vi "Delete Project Tasks.vi"(8 "error in (no error)":errorcluster, 9 "Tasks":string[](array[string]), 10 "Project Name":string, 11 "Projects in":refnum<class "Projects.lvclass">) -> (0 "error out":errorcluster, 2 "Success?":bool, 3 "Projects out":refnum<class "Projects.lvclass">)   [LabVIEW 2020, in "Projects.lvclass"]
doc: "Removes the Tasks from project indicated by Project Name. Success? will output True if the tasks are not present in the Project and the Project Name was a valid name.\n\n03/2025 Erich Schlieper"
uses:
  Projects.lvclass
  Projects.lvclass/Projects.ctl
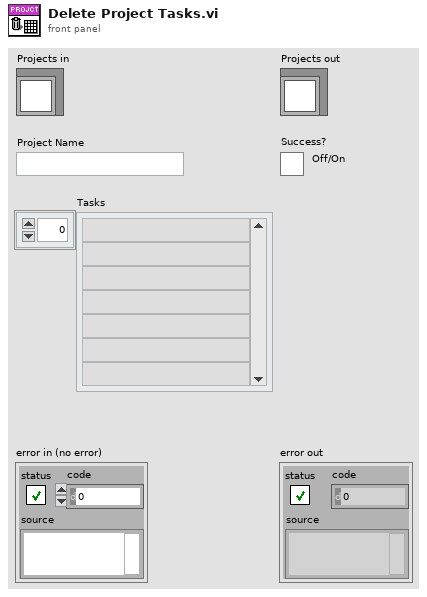
[diagram p1: front panel]
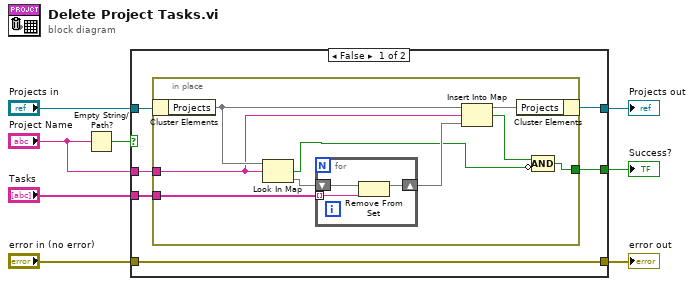
[diagram p0: block diagram]
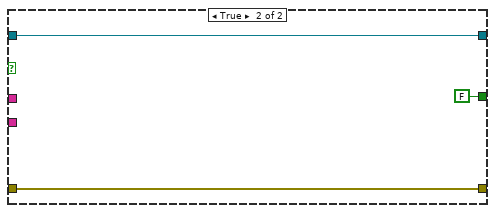
[diagram p2: hidden frame]
diagram:
  n1 = Empty String/Path?(string/path="Project Name") -> (empty?=w1:bool)
  n2 = case shown="False" w1 {
    tunnel: [w13 w29] -> w7
    tunnel: [w12 w28] -> w5
    tunnel: "Projects in" -> [w14 w28]
    tunnel: "Project Name" -> [w11 _]
    tunnel: "Tasks" -> [w10 _]
    tunnel: [w9 FALSE] -> w3
    tunnel: "error in (no error)" -> [w13 w29]
    frame False {
      n3 = in-place {
        in-place-border: w11 -> [w18]
        in-place-border: w10 -> [w22]
        in-place-border: [w15] -> w9
        n4 = in-place-cluster #1(w14) -> ("Projects"=w21:map{string, set{string}})
        n5 = Look In Map(map=w21, key=w18) -> (key not found?=w16:bool, value=w23:set{string})  [unwired: 1 in]
        n6 = for {
          shift-right: [w25] -> w19
          shift-left: w23 -> [w26]
          tunnel: w22 -> [w24] mode=indexing
          n7 = Remove From Set(10:w24, 11:w26) -> (3:w25:set{string})  [unwired: 1 out]
        }
        n8 = Insert Into Map(map in=w21, key=w18, value=w19) -> (map out=w20:map{string, set{string}}, key already included?=w17:bool)  [unwired: 1 out]
        n9 = in-place-cluster #1("Projects"=w20) -> (w12:refnum<class "Projects.lvclass">)
        n10 = Compound Arithmetic op=AND(w17, invert w16) -> (w15:bool)
      }
    }
    frame True {
    }
  }
  "error out" <- w7
  "Projects out" <- w5
  "Success?" <- w3
